vi "Acquisition Message Loop.vi"(8 "System Control":refnum<queue>, 10 "Instrument Manager":refnum<queue>, 11 "Acquisition":refnum<queue>) -> (0 "error out":errorcluster)   [LabVIEW 2020, in "ChromTech Next Gen Pump.lvlib" / "Acquisition.lvlib"]
doc: "Message loop for handling messages pertaining to the acquisition of data from the hardware."
uses:
  Acquisition.lvlib
  support/Message Queue/Message Cluster.ctl
  Acquisition State.ctl
  Hardware Configuration.ctl
  <vilib>/Utility/error.llb/Error Cluster From Error Code.vi
  <vilib>/ErrorRing/Error Ring.xnode
  support/Message Queue/Message Queue.lvlib
panel:
  in  "error in (no error)":errorcluster
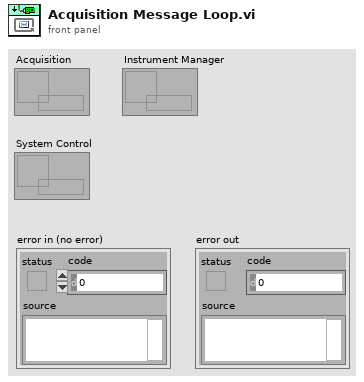
[diagram p1: front panel]
types:
  T1 = typedef "ChromTech Next Gen Pump.lvlib/Acquisition.lvlib/Hardware Configuration.ctl" = cluster{"Sample rate (sec/sample)":dbl, "Time Waited (sec)":dbl, "Acquisition Messages":string[]}
  T2 = typedef "ChromTech Next Gen Pump.lvlib/Acquisition.lvlib/Acquisition State.ctl" = enum16{"Idle", "Acquiring"}
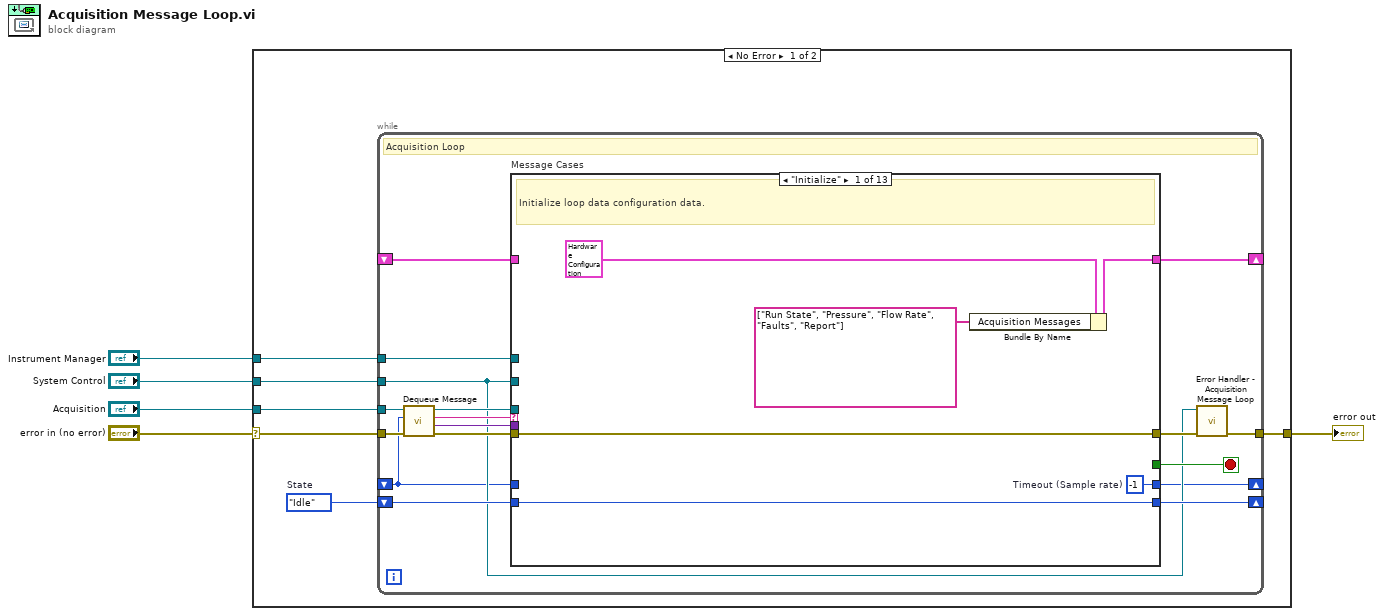
[diagram p0: block diagram]
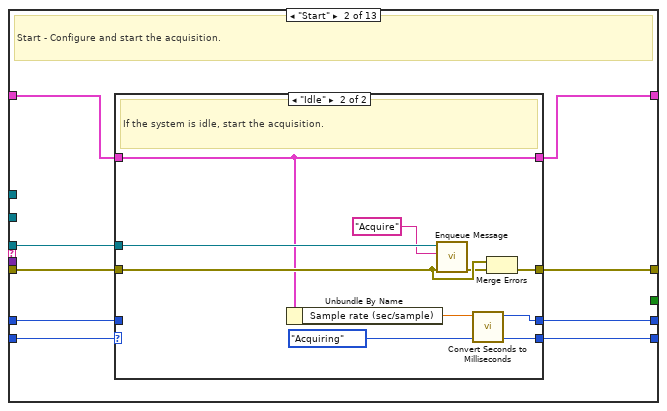
[diagram p2: hidden frame]
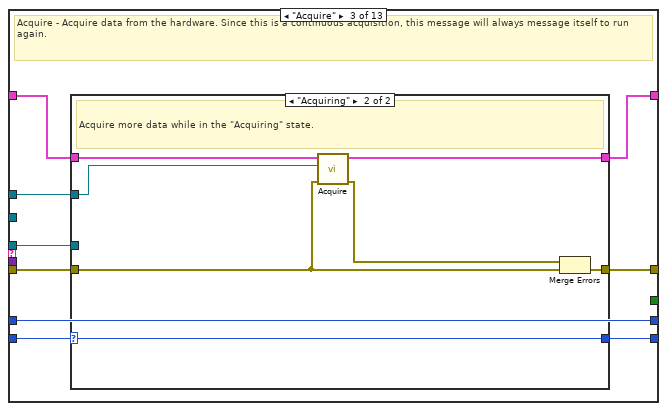
[diagram p4: hidden frame]
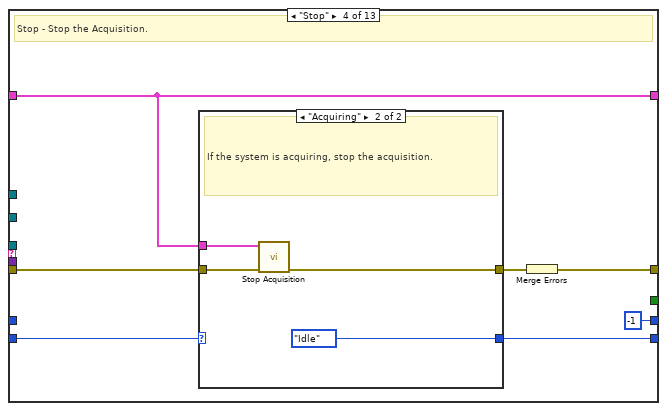
[diagram p6: hidden frame]
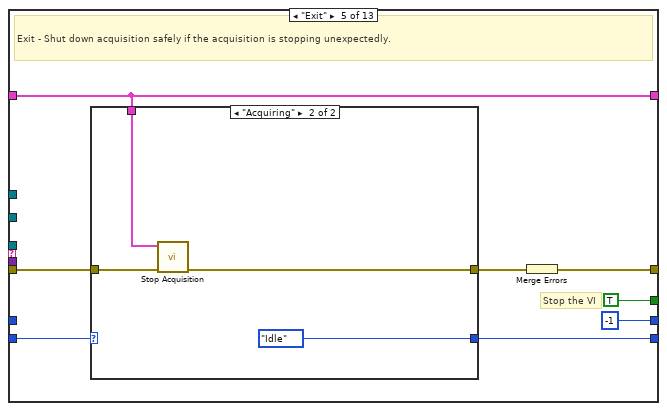
[diagram p8: hidden frame]
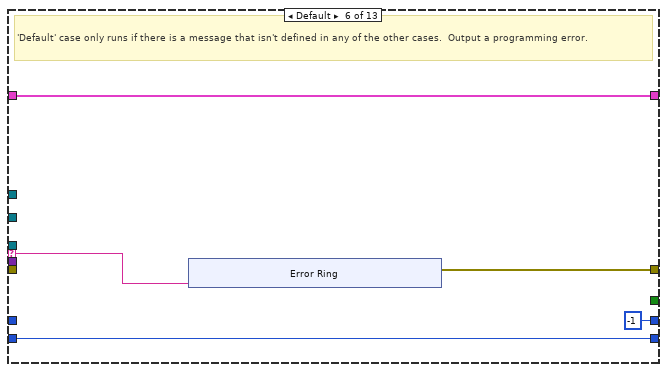
[diagram p10: hidden frame]
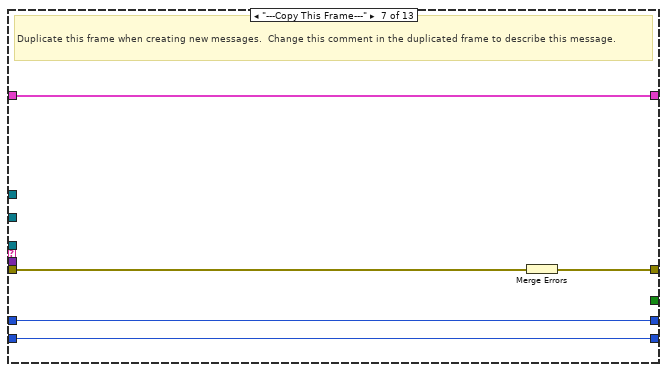
[diagram p11: hidden frame]
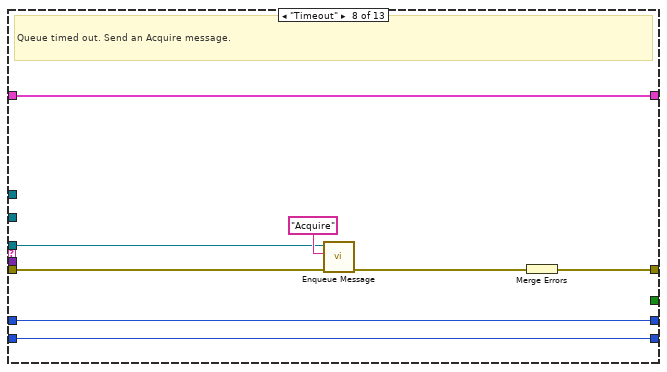
[diagram p12: hidden frame]
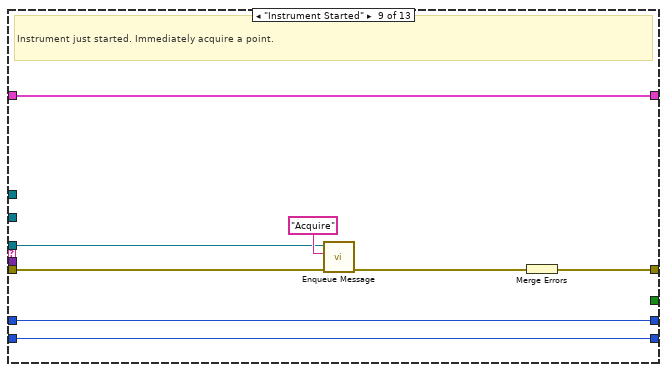
[diagram p13: hidden frame]
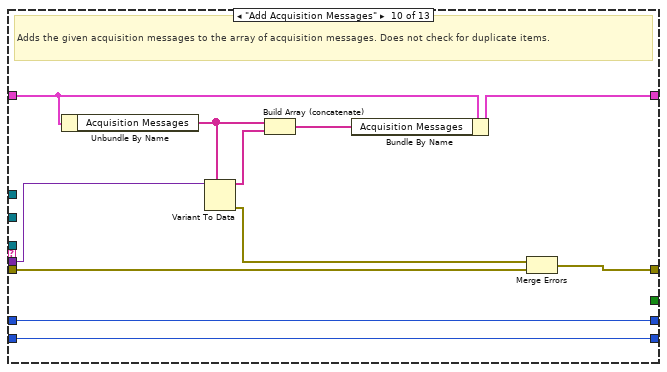
[diagram p14: hidden frame]
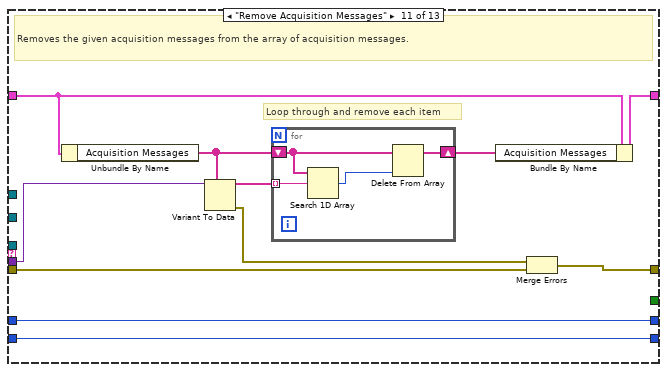
[diagram p15: hidden frame]
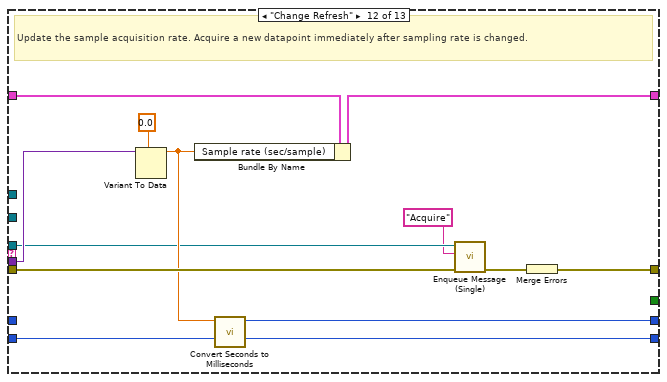
[diagram p16: hidden frame]
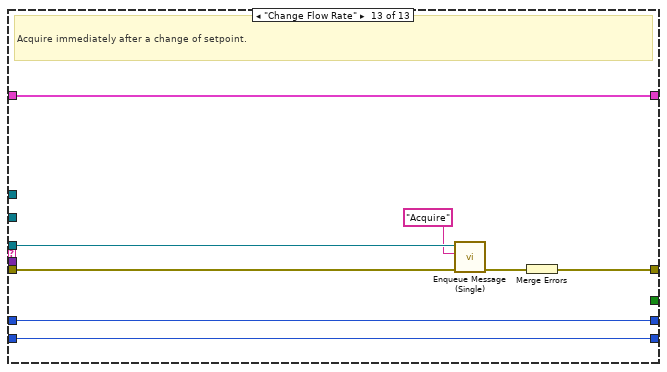
[diagram p17: hidden frame]
diagram:
  n1 = case shown="No Error" "error in (no error)" {
    selector: "error in (no error)" -> [w10 w182]
    tunnel: [w11 w182] -> w5
    tunnel: "Acquisition" -> [w8 _]
    tunnel: "System Control" -> [w7 _]
    tunnel: "Instrument Manager" -> [w6 _]
    frame No Error {
      w9 = Acquisition_State."Idle"  # State
      n2 = while {
        tunnel: w8 -> [w21]
        shift-right: [w27] -> _
        shift-left: _ -> [w28]
        tunnel: w7 -> [w15]
        shift-right: [w19] -> _
        shift-left: w9 -> [w20]
        tunnel: w10 -> [w25]
        tunnel: [w18] -> w11
        tunnel: w6 -> [w14]
        shift-right: [w13] -> _
        shift-left: _ -> [w12]
        stop <- w26 stop-if-true
        # "Acquisition Loop"
        n3 = call "Dequeue Message.vi"("error in (no error)"=w25, "timeout in ms (-1)"=w12, "Message Queue"=w21) -> ("error out"=w24:errorcluster, "Message Data"=w22:variant, "Message"=w23:string, "dup Message Queue"=w16:refnum<queue>)  [unwired: 5 in]
        n4 = case "Message Cases" shown="\"Initialize\"" w23 {
          selector: w23 -> [_ _ _ _ _ w104 _ _ _ _ _ _ _]
          tunnel: w16 -> [_ w40 w64 _ _ _ _ w120 w128 _ _ w163 w176]
          tunnel: w24 -> [w34 w41 w63 w81 w92 _ w119 w122 w130 w146 w157 w173 w181]
          tunnel: [w34 w43 w65 w82 w95 w105 w117 w126 w134 w145 w156 w171 w179] -> w17
          tunnel: w28 -> [_ w42 w61 w79 w90 w107 w118 w127 w135 w143 w154 w172 w180]
          tunnel: [w31 w39 w62 w79 w90 w107 w118 w127 w135 w138 w151 w169 w180] -> w27
          tunnel: [_ _ _ _ TRUE _ _ _ _ _ _ _ _] -> w26
          tunnel: w22 -> [_ _ _ _ _ _ _ _ _ w142 w153 w168 _]
          tunnel: w15 -> [_ _ _ _ _ _ _ _ _ _ _ _ _]
          tunnel: w20 -> [w33 w37 w59 w78 w94 w106 w116 w125 w133 w144 w155 w170 w178]
          tunnel: [w33 w38 w60 w77 w93 w106 w116 w125 w133 w144 w155 w170 w178] -> w19
          tunnel: w14 -> [_ _ w58 _ _ _ _ _ _ _ _ _ _]
          tunnel: [w29 w36 w57 -1 ("Time (ms)") -1 ("Time (ms)") -1 ("Time (ms)") w115 w124 w132 w136 w147 w165 w174] -> w13
          tunnel: w12 -> [_ w35 w57 _ _ _ w115 w124 w132 w136 w147 _ w174]
          frame "Initialize" {
            w29 = -1  # Timeout (Sample rate)
            # "Initialize loop data configuration data."
            n5 = Bundle By Name(cluster=T1 {"Sample rate (sec/sample)"=5.0, "Time Waited (sec)"=0.0, "Acquisition Messages"=["Run State", "Example Value <Replace Me>", "Setpoint", "Report"]} ("Acquisition Configuration"), "Acquisition Messages"=string[] ["Run State", "Pressure", "Flow Rate", "Faults", "Report"]) -> (w31:T1)
          }
          frame "Start" {
            # "Start - Configure and start the acquisition."
            n6 = case shown="\"Idle\"" w37 {
              selector: w37 -> [w45 _]
              tunnel: [w46 w56] -> w43
              tunnel: w42 -> [w47 w50]
              tunnel: w41 -> [w46 w55]
              tunnel: w40 -> [_ w53]
              tunnel: [w47 w50] -> w39
              tunnel: [w45 Acquisition_State."Acquiring" ("Acquisition State")] -> w38
              tunnel: [w44 w48] -> w36
              tunnel: w35 -> [w44 _]
              frame "Acquiring" {
                # "The system is already acquiring. Ignore the \"Start\" message."
              }
              frame "Idle" {
                # "If the system is idle, start the acquisition."
                n7 = Unbundle By Name(w50) -> ("Sample rate (sec/sample)"=w49:dbl)
                n8 = call-poly "Enqueue Message.vi"("error in (no error)"=w55, "Message"="Acquire", "Message Queue"=w53) -> ("error out"=w54:errorcluster)  [unwired: 7 in, 1 out]
                n9 = call "Convert Seconds to Milliseconds.vi"("Time (sec)"=w49) -> ("Time (ms)"=w48:i32)  [unwired: 10 in]
                n10 = Merge Errors(w55, w54) -> (w56:errorcluster)
              }
            }
          }
          frame "Acquire" {
            # "Acquire - Acquire data from the hardware. Since this is a continuous acquisition, this message will always message itself to run again."
            n11 = case shown="\"Acquiring\"" w59 {
              selector: w59 -> [w66 w73]
              tunnel: [w67 w75] -> w65
              tunnel: w64 -> [_ _]
              tunnel: w63 -> [w67 w72]
              tunnel: [w68 w69] -> w62
              tunnel: w61 -> [w68 w71]
              tunnel: [w66 w73] -> w60
              tunnel: w58 -> [_ w70]
              frame "Idle" {
                # "Ignore \"Acquire\" messages when the acquisition is idle."
              }
              frame "Acquiring" {
                # "Acquire more data while in the \"Acquiring\" state."
                n12 = call "Acquire.vi"("error in (no error)"=w72, "Instrument Manager"=w70, "Acquisition Config in"=w71) -> ("error out"=w74:errorcluster, "Acquisition Config out (dup)"=w69:T1)  [unwired: 7 in]
                n13 = Merge Errors(w74, w72) -> (w75:errorcluster)
              }
            }
          }
          frame "Stop" {
            # "Stop - Stop the Acquisition."
            n14 = case shown="\"Acquiring\"" w78 {
              selector: w78 -> [w83 _]
              tunnel: w81 -> [w84 w88]
              tunnel: [w84 w87] -> w80
              tunnel: w79 -> [_ w86]
              tunnel: [w83 Acquisition_State."Idle" ("State")] -> w77
              frame "Idle" {
                # "The system is already idle. Ignore the \"Stop\" message."
              }
              frame "Acquiring" {
                # "If the system is acquiring, stop the acquisition."
                n15 = call "Stop Acquisition.vi"("error in (no error)"=w88, "Acquisition Configuration in"=w86) -> ("error out"=w87:errorcluster)  [unwired: 9 in]
              }
            }
            n16 = Merge Errors(w80) -> (w82:errorcluster)
          }
          frame "Exit" {
            # "Stop the VI"
            # "Exit - Shut down acquisition safely if the acquisition is stopping unexpectedly."
            n17 = case shown="\"Acquiring\"" w94 {
              selector: w94 -> [w98 _]
              tunnel: [w98 Acquisition_State."Idle" ("State")] -> w93
              tunnel: w92 -> [w97 w101]
              tunnel: [w97 w100] -> w91
              tunnel: w90 -> [_ w99]
              frame "Idle", Default {
              }
              frame "Acquiring" {
                n18 = call "Stop Acquisition.vi"("error in (no error)"=w101, "Acquisition Configuration in"=w99) -> ("error out"=w100:errorcluster)  [unwired: 9 in]
              }
            }
            n19 = Merge Errors(w91) -> (w95:errorcluster)
          }
          frame Default {
            # "'Default' case only runs if there is a message that isn't defined in any of the other cases.  Output a programming error."
            n20 = xnode "Error Ring"("parameter 0"=w104) -> ("error out"=w105:errorcluster)
          }
          frame "---Copy This Frame---" {
            # "Duplicate this frame when creating new messages.  Change this comment in the duplicated frame to describe this message."
            n21 = Merge Errors(w119) -> (w117:errorcluster)
          }
          frame "Timeout" {
            # "Queue timed out. Send an Acquire message."
            n22 = call-poly "Enqueue Message.vi"("error in (no error)"=w122, "Message"="Acquire", "Message Queue"=w120) -> ("error out"=w121:errorcluster)  [unwired: 7 in, 1 out]
            n23 = Merge Errors(w121) -> (w126:errorcluster)
          }
          frame "Instrument Started" {
            # "Instrument just started. Immediately acquire a point."
            n24 = call-poly "Enqueue Message.vi"("error in (no error)"=w130, "Message"="Acquire", "Message Queue"=w128) -> ("error out"=w129:errorcluster)  [unwired: 7 in, 1 out]
            n25 = Merge Errors(w129) -> (w134:errorcluster)
          }
          frame "Add Acquisition Messages" {
            # "Adds the given acquisition messages to the array of acquisition messages. Does not check for duplicate items."
            n26 = Unbundle By Name(w143) -> ("Acquisition Messages"=w140:string[])
            n27 = Variant To Data(type=w140, Variant=w142) -> (data=w139:string[], error out=w141:errorcluster)  [unwired: 1 in]
            n28 = Build Array (concatenate)(w140, w139) -> (w137:string[])
            n29 = Bundle By Name(cluster=w143, "Acquisition Messages"=w137) -> (w138:T1)
            n30 = Merge Errors(w141, w146) -> (w145:errorcluster)
          }
          frame "Remove Acquisition Messages" {
            # "Loop through and remove each item"
            # "Removes the given acquisition messages from the array of acquisition messages."
            n31 = Unbundle By Name(w154) -> ("Acquisition Messages"=w149:string[])
            n32 = Variant To Data(type=w149, Variant=w153) -> (data=w150:string[], error out=w152:errorcluster)  [unwired: 1 in]
            n33 = for {
              tunnel: w150 -> [w161] mode=indexing
              shift-right: [w158] -> w148
              shift-left: w149 -> [w159]
              n34 = Search 1D Array(1D array=w159, element=w161) -> (index of element=w160:i32)  [unwired: 1 in]
              n35 = Delete From Array(array=w159, index=w160) -> (array with subset deleted=w158:string[])  [unwired: 1 in, 1 out]
            }
            n36 = Bundle By Name(cluster=w154, "Acquisition Messages"=w148) -> (w151:T1)
            n37 = Merge Errors(w152, w157) -> (w156:errorcluster)
          }
          frame "Change Refresh" {
            # "Update the sample acquisition rate. Acquire a new datapoint immediately after sampling rate is changed."
            n38 = Variant To Data(type=0.0 ("Hardware Reference"), Variant=w168) -> (data=w166:dbl)  [unwired: 1 in, 1 out]
            n39 = Bundle By Name(cluster=w172, "Sample rate (sec/sample)"=w166) -> (w169:T1)
            n40 = call "Convert Seconds to Milliseconds.vi"("Time (sec)"=w166) -> ("Time (ms)"=w165:i32)  [unwired: 10 in]
            n41 = call "Enqueue Message (Single).vi"("error in (no error)"=w173, "Message"="Acquire", "Message Queue"=w163) -> ("error out"=w164:errorcluster)  [unwired: 7 in, 1 out]
            n42 = Merge Errors(w164) -> (w171:errorcluster)
          }
          frame "Change Flow Rate" {
            # "Acquire immediately after a change of setpoint."
            n43 = call "Enqueue Message (Single).vi"("error in (no error)"=w181, "Message"="Acquire", "Message Queue"=w176) -> ("error out"=w177:errorcluster)  [unwired: 7 in, 1 out]
            n44 = Merge Errors(w177) -> (w179:errorcluster)
          }
        }
        n45 = call "Error Handler - Acquisition Message Loop.vi"("error in (no error)"=w17, "Message Queue"=w15) -> ("dup error in"=w18:errorcluster)  [unwired: 8 in, 1 out]
      }
    }
    frame Error {
    }
  }
  "error out" <- w5
